vi "CopyImageNoMaskARGB.vi"(8 "error in (no error)":errorcluster, 10 "ARGB Image Destination":refnum<data-value>, 11 "ARGB Image Source":refnum<data-value>) -> (0 "error out":errorcluster, 3 "ARGB Image Destination (duplicate)":refnum<data-value>)   [LabVIEW 2020, in "g_ar_toolkit.image.lvlib"]
uses:
  g_ar_toolkit.image.lvlib
  d58821cd-5760-454c-8714-6bb79b1811ae.vi
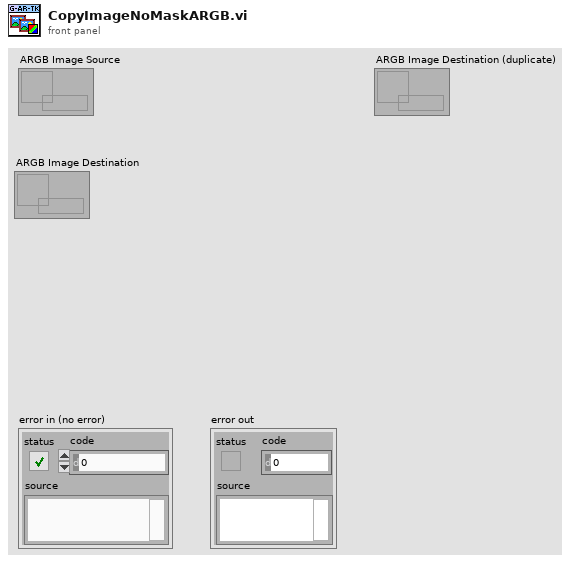
[diagram p1: front panel]
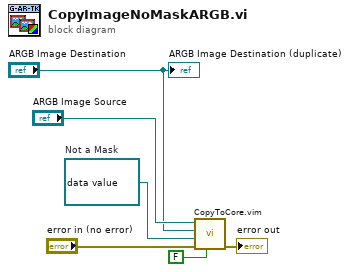
[diagram p0: block diagram]
diagram:
  w3 = refnum<data-value> refnum  # Not a Mask
  n1 = call "CopyToCore.vim"("Has Mask"=FALSE, "error in (no error)"="error in (no error)", "Mask"=w3, "Dst"="ARGB Image Destination", "Src"="ARGB Image Source") -> ("error out"=→"error out":errorcluster)  [unwired: 6 in]
  "ARGB Image Destination (duplicate)" <- "ARGB Image Destination"
